vi "GetFiltDataFilesNm.vi"(6 "IncludeSubF":bool, 8 "error in (no error)":errorcluster, 9 "Session":i32=-1, 10 "Date String":string="All" caption="Date String (yymmdd or All or Range)", 11 "Data Folder Path":path) -> (0 "error out":errorcluster, 3 "HdrFilesNames":path[](array[path]))   [LabVIEW 2012]
panel:
  out "valeur sélectionnée":string
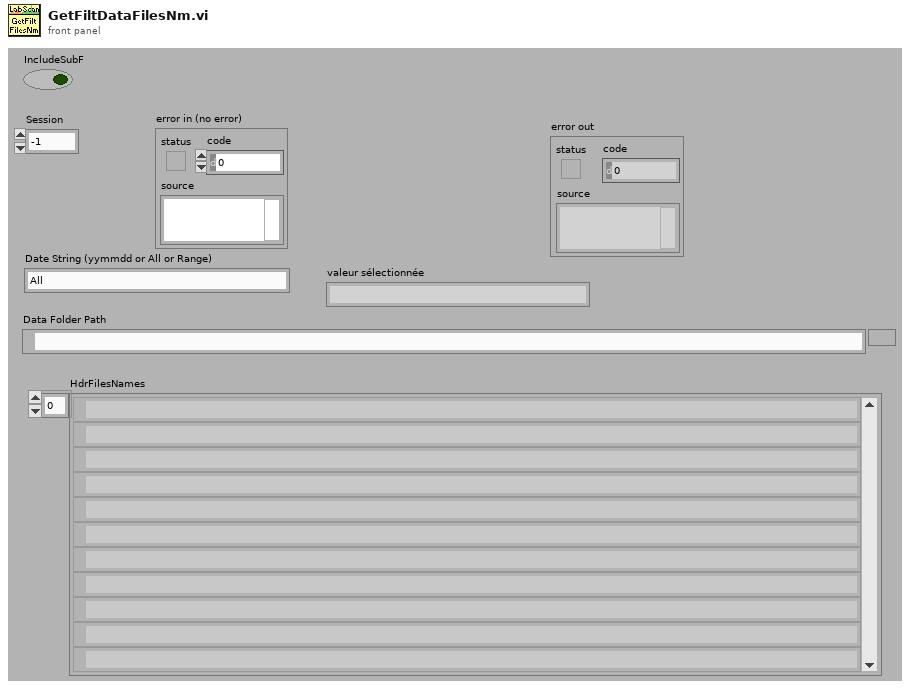
[diagram p1: front panel]
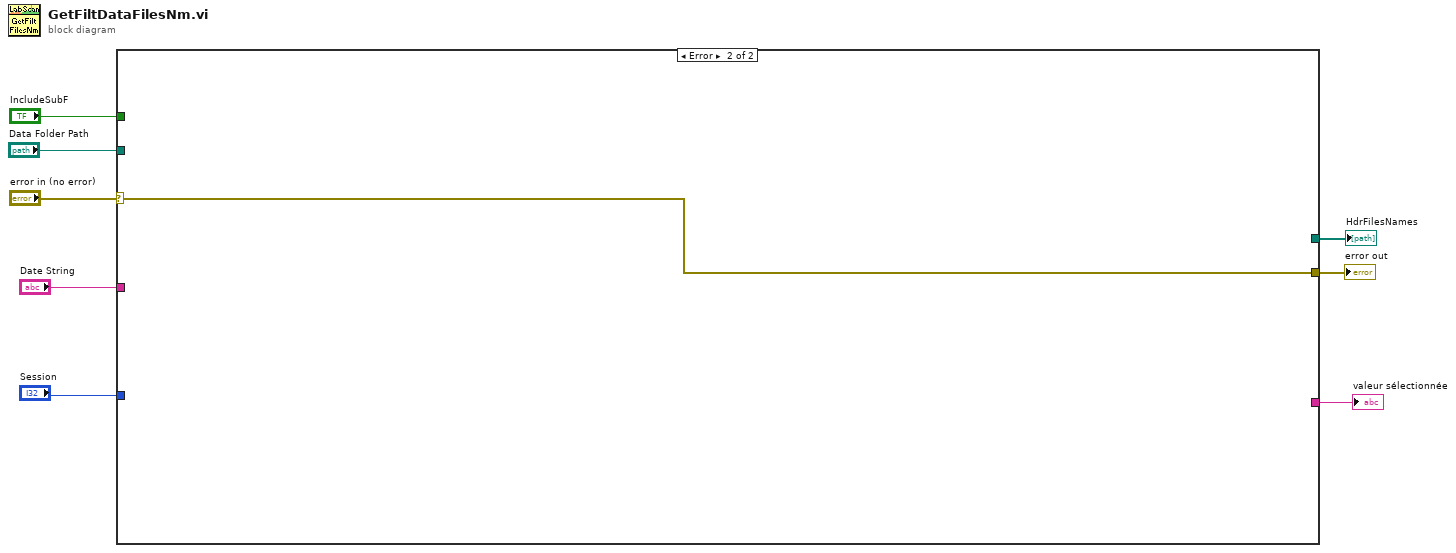
[diagram p0: block diagram]
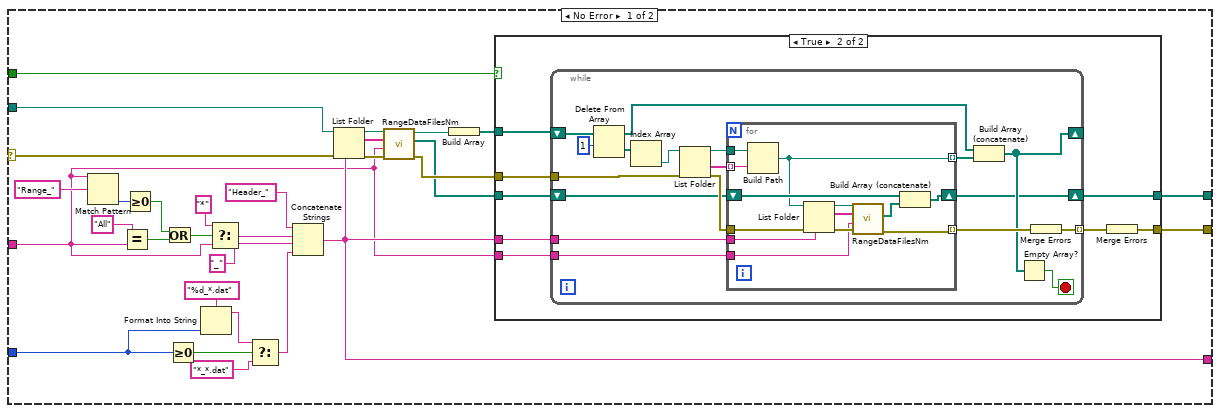
[diagram p2: hidden frame]
diagram:
  n1 = case shown="Error" "error in (no error)" {
    selector: "error in (no error)" -> [w9 w80]
    tunnel: "Session" -> [w34 _]
    tunnel: [w25 w80] -> w7
    tunnel: "IncludeSubF" -> [w24 _]
    tunnel: [w23 _] -> w5
    tunnel: "Date String" -> [w14 _]
    tunnel: "Data Folder Path" -> [w13 _]
    tunnel: [w10 _] -> w2
    frame No Error {
      n2 = Match Pattern(string=w14, regular expression="Range_" ("chaîne de format")) -> (offset past match=w20:i32)  [unwired: 1 in, 3 out]
      n3 = Equal?(x="All" ("Date String"), y=w14) -> (x = y?=w33:bool)
      n4 = Greater Or Equal To 0?(x=w20) -> (x >= 0?=w19:bool)
      n5 = Or(x=w19, y=w33) -> (x .or. y?=w26:bool)
      n6 = Greater Or Equal To 0?(x=w34) -> (x >= 0?=w38:bool)
      n7 = Format Into String(format string="%d_*.dat" ("filtre"), w34) -> (resulting string=w36:string)  [unwired: 2 in, 1 out]
      n8 = Select(t="*", s=w26, f=w14) -> (s? t:f=w31:string)
      n9 = Select(t=w36, s=w38, f="*_*.dat" ("filtre")) -> (s? t:f=w29:string)
      n10 = Concatenate Strings("Header_", w31, "_" ("filtre"), w29) -> (w23:string)
      n11 = List Folder(path=w13, pattern=w23, error in=w9) -> (path out=w18:path, filenames=w17:string[], error out=w16:errorcluster)  [unwired: 1 in, 1 out]
      n12 = call "RangeDataFilesNm.vi"("error in (no error)"=w16, "Range_String"=w14, "noms des fichiers"=w17, "DataPath"=w18) -> ("error out"=w15:errorcluster, "HdrFilesNames"=w12:path[], "DataPathOut"=w11:path)  [unwired: 5 in]
      n13 = Build Array(w11) -> (w22:path[])
      n14 = case shown="True" w24 {
        tunnel: w22 -> [_ w45]
        tunnel: w12 -> [w40 w48]
        tunnel: [w40 w43] -> w10
        tunnel: w15 -> [w39 w44]
        tunnel: [w39 w42] -> w25
        tunnel: w23 -> [_ w46]
        tunnel: w14 -> [_ w41]
        frame False {
        }
        frame True {
          n15 = while {
            tunnel: [w65] -> w47 mode=indexing
            tunnel: w46 -> [w64]
            tunnel: w44 -> [w62]
            shift-right: [w53] -> _
            shift-left: w45 -> [w59]
            shift-right: [w50] -> w43
            shift-left: w48 -> [w51]
            tunnel: w41 -> [w49]
            stop <- w52 stop-if-true
            n16 = Delete From Array(array=w59, length=1 ("longueur")) -> (deleted portion=w55:path[], array with subset deleted=w57:path[])  [unwired: 1 in]
            n17 = Index Array(array=w55) -> (element=w54:path)  [unwired: 1 in]
            n18 = List Folder(path=w54, error in=w62) -> (path out=w60:path, folder names=w63:string[], error out=w61:errorcluster)  [unwired: 2 in, 1 out]
            n19 = for {
              tunnel: w63 -> [w79] mode=indexing
              tunnel: w60 -> [w78]
              shift-right: [w68] -> w50
              shift-left: w51 -> [w77]
              tunnel: w61 -> [w76]
              tunnel: [w72] -> w66 mode=indexing
              tunnel: w64 -> [w75]
              tunnel: [w74] -> w56 mode=indexing
              tunnel: w49 -> [w69]
              n20 = Build Path(base path=w78, name or relative path=w79) -> (appended path=w74:path)
              n21 = List Folder(path=w74, pattern=w75, error in=w76) -> (path out=w71:path, filenames=w70:string[], error out=w73:errorcluster)  [unwired: 1 in, 1 out]
              n22 = call "RangeDataFilesNm.vi"("error in (no error)"=w73, "Range_String"=w69, "noms des fichiers"=w70, "DataPath"=w71) -> ("error out"=w72:errorcluster, "HdrFilesNames"=w67:path[])  [unwired: 5 in, 1 out]
              n23 = Build Array (concatenate)(w77, w67) -> (w68:path[])
            }
            n24 = Build Array (concatenate)(w57, w56) -> (w53:path[])
            n25 = Empty Array?(array=w53) -> (empty?=w52:bool)
            n26 = Merge Errors(w66) -> (w65:errorcluster)
          }
          n27 = Merge Errors(w47) -> (w42:errorcluster)
        }
      }
    }
    frame Error {
    }
  }
  "error out" <- w7
  "valeur sélectionnée" <- w5
  "HdrFilesNames" <- w2
